vi "Read TDMS Wavenames.vi"(8 "error in (no error)":errorcluster, 10 "path":path, 11 "LVtoITX in":refnum<class "LV to ITX.lvclass">) -> (0 "error out":errorcluster, 2 "Wavenames":string[](array[string]), 3 "LVtoITX out":refnum<class "LV to ITX.lvclass">)   [LabVIEW 2016, in "LV to ITX.lvclass"]
uses:
  LV to ITX.lvclass
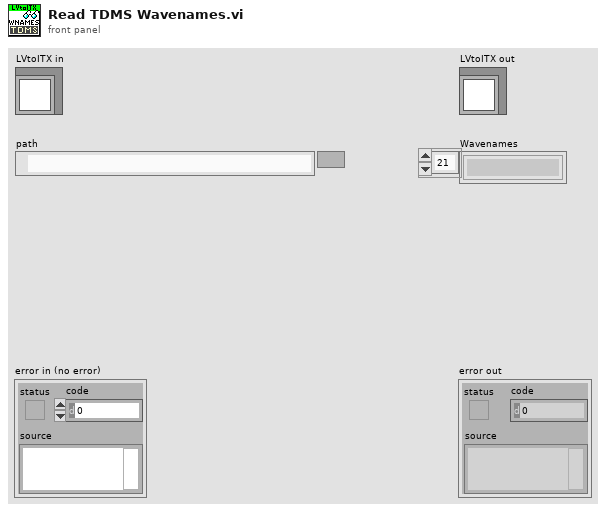
[diagram p1: front panel]
types:
  T1 = enum16{"open", "open or create", "create or replace", "create", "open (read-only)"}
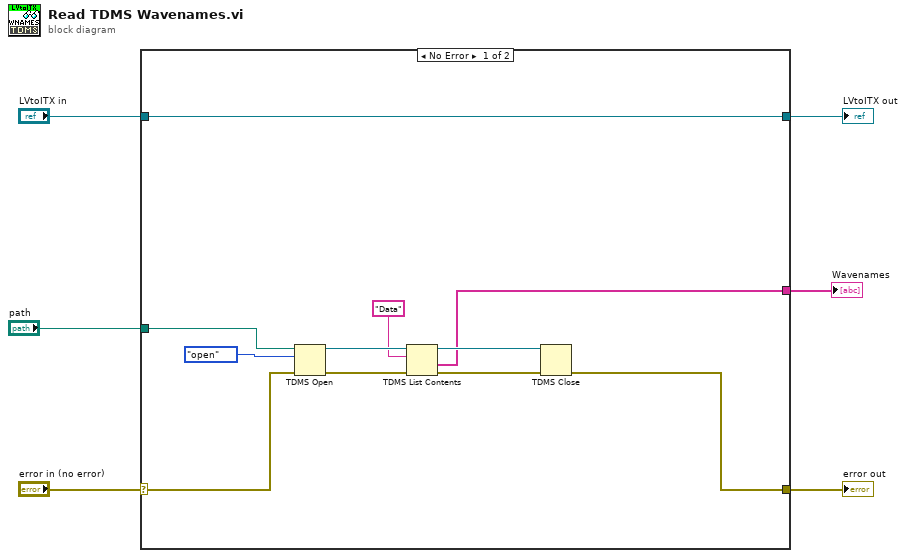
[diagram p0: block diagram]
diagram:
  n1 = case shown="No Error" "error in (no error)" {
    selector: "error in (no error)" -> [w9 w18]
    tunnel: [w14 w18] -> w3
    tunnel: [w8 w19] -> w4
    tunnel: "LVtoITX in" -> [w8 w19]
    tunnel: "path" -> [w12 _]
    tunnel: [w7 _] -> w1
    frame No Error {
      n2 = TDMS Open(8:w9, 10:T1."open" ("operation (0:open)"), 11:w12) -> (0:w15:errorcluster, 3:w16:refnum<k34>)  [unwired: 4 in]
      n3 = TDMS List Contents(4:w15, 6:"Data" ("group name"), 7:w16) -> (0:w11:errorcluster, 1:w7:string[], 3:w10:refnum<k34>)  [unwired: 1 out]
      n4 = TDMS Close(8:w11, 11:w10) -> (0:w14:errorcluster)  [unwired: 1 out]
    }
    frame Error {
    }
  }
  "error out" <- w3
  "LVtoITX out" <- w4
  "Wavenames" <- w1
